vi "client.vi"() -> ()   [LabVIEW 2019]
uses:
  <vilib>/httpClient/LabVIEWHTTPClient.lvlib
panel:
  out "value":cluster{"a":dbl, "b":dbl, "SUM":dbl}
  out "returned body":string
  out "returned headers":string
  in  "endpoint URL":string
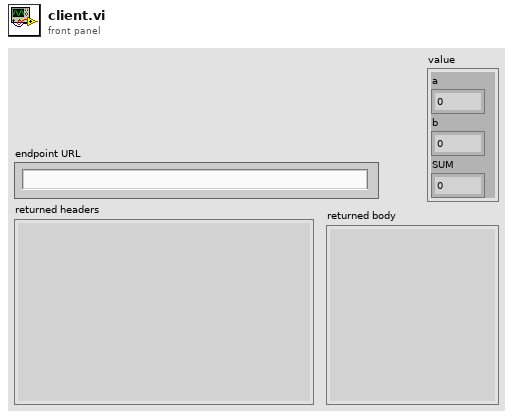
[diagram p1: front panel]
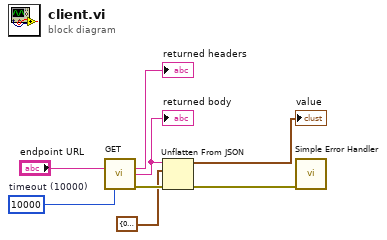
[diagram p0: block diagram]
diagram:
  w8 = 10000  # timeout (10000)
  n1 = call <vilib>:"GET.vi"("url"="endpoint URL", "timeout (10000)"=w8) -> ("headers"=→"returned headers":string, "body"=w5:string, "error out"=w4:errorcluster)  [unwired: 10 in, 1 out]
  "returned body" <- w5
  n2 = Unflatten From JSON(JSON string=w5, type and defaults=cluster{"a":dbl, "b":dbl, "SUM":dbl} {"a"=0.0, "b"=0.0, "SUM"=0.0} ("Cluster"), error in (no error)=w4) -> (value=→"value":cluster{"a":dbl, "b":dbl, "SUM":dbl}, error out=w3:errorcluster)  [unwired: 4 in]
  n3 = call <vilib>:"Simple Error Handler.vi"("error in (no error)"=w3) -> ()  [unwired: 4 in, 5 out]
